vi "Pulse Generator- user input.vi"() -> ()   [LabVIEW 2020]
uses:
  <vilib>/DAQmx/create/channels.llb/DAQmx Create Channel (CO-Pulse Generation-Frequency).vi
  <vilib>/DAQmx/configure/timing.llb/DAQmx Timing (Implicit).vi
  <resource>/objmgr/daqmx.rc
panel:
  out "Output Duty Cycle":dbl
  in  "Duty Cycle":dbl(slide)=0.01 min=0.01 max=0.99 scale=0.01..0.99
  in  "Output Pulse":tag
  out "Output Frequency":dbl
  in  "counter":tag
  in  "stop":bool
  in  "Input Frequency":dbl=1.0 min=1.0 max=25000000.0 step=1000.0
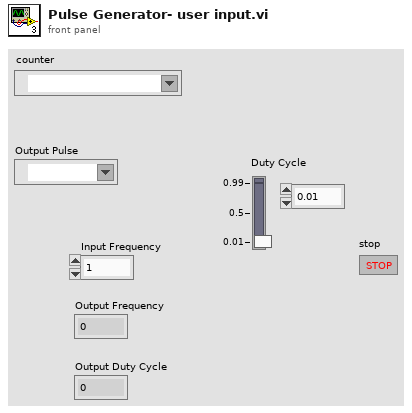
[diagram p1: front panel]
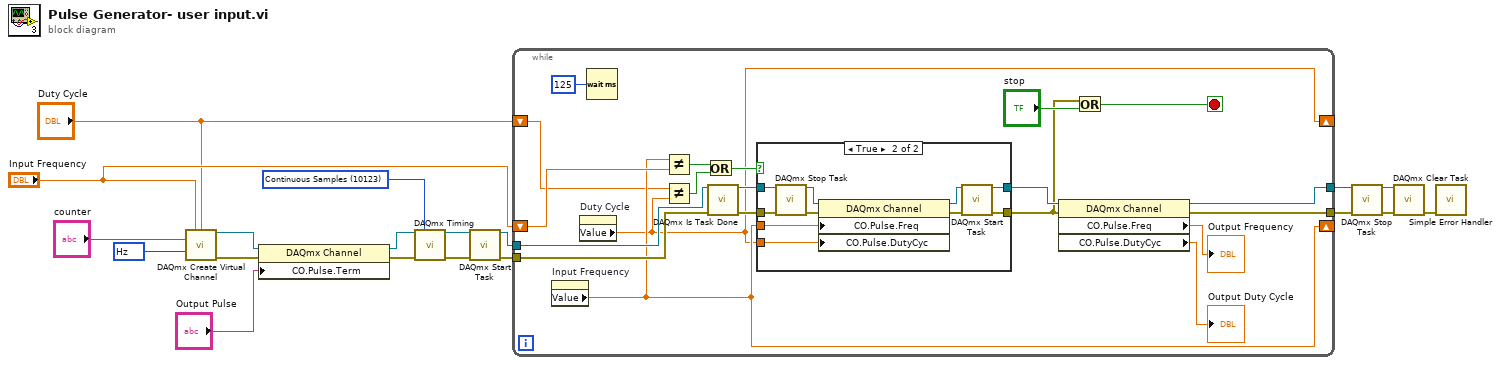
[diagram p0: block diagram]
diagram:
  w18 = 10123 items=["Finite Samples"=10178, "Continuous Samples"=10123, "Hardware Timed Single Point"=12522] ("sample mode")
  w19 = 10373 items=["Hz"=10373] ("units")
  n1 = call-poly <vilib>:"DAQmx Create Virtual Channel.vi"("frequency"="Input Frequency", "duty cycle"="Duty Cycle", "counter"="counter", "units"=w19) -> ("task out"=w6:refnum<k21>, "error out"=w5:errorcluster)  [unwired: 10 in]
  n2 = property class="DAQmx Channel"(reference=w6, error in=w5, "CO.Pulse.Term"="Output Pulse") -> (reference out=w4:refnum<k21>, error out=w3:errorcluster)
  n3 = call-poly <vilib>:"DAQmx Timing.vi"("task/channels in"=w4, "sample mode"=w18, "error in"=w3) -> ("task out"=w17:refnum<k21>, "error out"=w16:errorcluster)  [unwired: 11 in]
  n4 = call <vilib>:"DAQmx Start Task.vi"("task/channels in"=w17, "error in"=w16) -> ("task out"=w15:refnum<k21>, "error out"=w14:errorcluster)  [unwired: 12 in]
  n5 = while {
    tunnel: w15 -> [w39]
    tunnel: w14 -> [w38]
    shift-right: [w29] -> _
    shift-left: "Input Frequency" -> [w33]
    tunnel: [w28] -> w8
    tunnel: [w27] -> w7
    shift-right: [w22] -> _
    shift-left: "Duty Cycle" -> [w23]
    stop <- w35 stop-if-true
    n6 = property on="Input Frequency" class="DigNum (strict)"() -> ("Value"=w29:dbl)  [unwired: 2 in, 2 out]
    n7 = property on="Duty Cycle" class="Slide (strict)"() -> ("Value"=w22:dbl)  [unwired: 2 in, 2 out]
    n8 = Wait (ms)(milliseconds to wait=u32 125) -> ()  [unwired: 1 out]
    n9 = Not Equal?(x=w29, y=w33) -> (x != y?=w24:bool)
    n10 = Not Equal?(x=w23, y=w22) -> (x != y?=w20:bool)
    n11 = Or(x=w24, y=w20) -> (x .or. y?=w25:bool)
    n12 = call <vilib>:"DAQmx Is Task Done.vi"("task/channels in"=w39, "error in"=w38) -> ("task out"=w37:refnum<k21>, "error out"=w36:errorcluster)  [unwired: 11 in, 1 out]
    n13 = case shown="True" w25 {
      tunnel: w37 -> [w41 w50]
      tunnel: w36 -> [w40 w49]
      tunnel: w29 -> [_ w51]
      tunnel: [w41 w46] -> w31
      tunnel: [w40 w45] -> w21
      tunnel: w22 -> [_ w42]
      frame False {
      }
      frame True {
        n14 = call <vilib>:"DAQmx Stop Task.vi"("task/channels in"=w50, "error in"=w49) -> ("task out"=w48:refnum<k21>, "error out"=w47:errorcluster)  [unwired: 12 in]
        n15 = property class="DAQmx Channel"(reference=w48, error in=w47, "CO.Pulse.Freq"=w51, "CO.Pulse.DutyCyc"=w42) -> (reference out=w43:refnum<k21>, error out=w44:errorcluster)
        n16 = call <vilib>:"DAQmx Start Task.vi"("task/channels in"=w43, "error in"=w44) -> ("task out"=w46:refnum<k21>, "error out"=w45:errorcluster)  [unwired: 12 in]
      }
    }
    n17 = property class="DAQmx Channel"(reference=w31, error in=w21) -> (reference out=w28:refnum<k21>, error out=w27:errorcluster, "CO.Pulse.Freq"=→"Output Frequency":dbl, "CO.Pulse.DutyCyc"=→"Output Duty Cycle":dbl)
    n18 = Or(x=w21, y="stop") -> (x .or. y?=w35:bool)
  }
  n19 = call <vilib>:"DAQmx Stop Task.vi"("task/channels in"=w8, "error in"=w7) -> ("task out"=w12:refnum<k21>, "error out"=w11:errorcluster)  [unwired: 12 in]
  n20 = call <vilib>:"DAQmx Clear Task.vi"("task in"=w12, "error in"=w11) -> ("error out"=w10:errorcluster)  [unwired: 13 in]
  n21 = call <vilib>:"Simple Error Handler.vi"("error in (no error)"=w10) -> ()  [unwired: 4 in, 5 out]
